vi "RPT_Convert Results.vi"(9 "disabled index (col)":i32, 10 "Results IN":T1 {"Resistor 2" format="%.1f"; "Drain" format="%.3f"; "Resistor" format="%.1f"; "Fill" format="%.3f"}) -> (2 "Report OUt":string[][](array[string]), 3 "ATP Table":string[][](array[string]))   [LabVIEW 2024]
uses:
  Control Definitions/Def Results3.ctl
  Control Definitions/Def_ATPStatus.ctl
  Control Definitions/Def Results.ctl
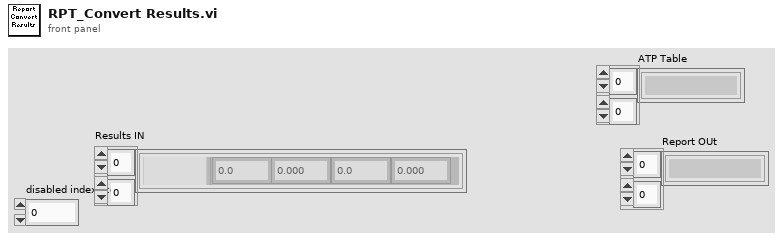
[diagram p1: front panel]
types:
  T1 = typedef "Def Results.ctl" = T2[][]
  T2 = typedef "Def Results3.ctl" = cluster{"Fill":dbl, "Status":T3, "Resistor":dbl, "Drain":dbl, "Resistor 2":dbl}
  T3 = typedef "Def_ATPStatus.ctl" = i16
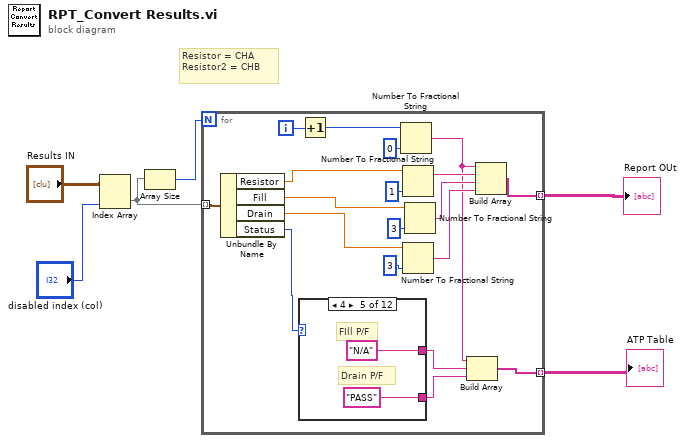
[diagram p0: block diagram]
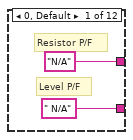
[diagram p2: hidden frame]
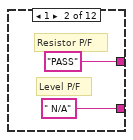
[diagram p3: hidden frame]
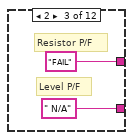
[diagram p4: hidden frame]
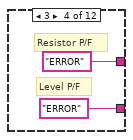
[diagram p5: hidden frame]
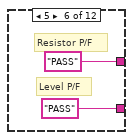
[diagram p6: hidden frame]
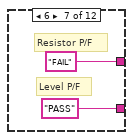
[diagram p7: hidden frame]
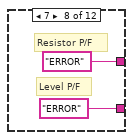
[diagram p8: hidden frame]
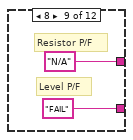
[diagram p9: hidden frame]
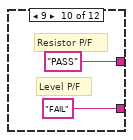
[diagram p10: hidden frame]
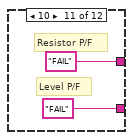
[diagram p11: hidden frame]
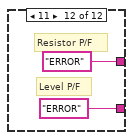
[diagram p12: hidden frame]
diagram:
  # "Resistor = CHA\nResistor2 = CHB"
  n1 = Index Array(array="Results IN", index (col)="disabled index (col)") -> (element=w5:T2[])  [unwired: 1 in]
  n2 = Array Size(array=w5) -> (size(s)=w4:i32)
  n3 = for {
    N: w4 -> [_]
    tunnel: w5 -> [w15] mode=indexing
    tunnel: [w19] -> w6 mode=indexing
    tunnel: [w8] -> w1 mode=indexing
    i -> [w18]
    n4 = Unbundle By Name(w15) -> ("Resistor"=w14:dbl, "Fill"=w13:dbl, "Drain"=w12:dbl, "Status"=w11:T3)
    n5 = case shown="4" w11 {
      tunnel: ["N/A" "PASS" "FAIL" "ERROR" "N/A" "PASS" "FAIL" "ERROR" "N/A" "PASS" "FAIL" "ERROR"] -> w10
      tunnel: [" N/A" " N/A" " N/A" "ERROR" "PASS" "PASS" "PASS" "ERROR" "FAIL" "FAIL" "FAIL" "ERROR"] -> w9
      frame 0, Default {
        # "Resistor P/F"
        # "Level P/F"
      }
      frame 1 {
        # "Resistor P/F"
        # "Level P/F"
      }
      frame 2 {
        # "Resistor P/F"
        # "Level P/F"
      }
      frame 3 {
        # "Resistor P/F"
        # "Level P/F"
      }
      frame 4 {
        # "FIll P/F"
        # "Drain P/F"
      }
      frame 5 {
        # "Resistor P/F"
        # "Level P/F"
      }
      frame 6 {
        # "Resistor P/F"
        # "Level P/F"
      }
      frame 7 {
        # "Resistor P/F"
        # "Level P/F"
      }
      frame 8 {
        # "Resistor P/F"
        # "Level P/F"
      }
      frame 9 {
        # "Resistor P/F"
        # "Level P/F"
      }
      frame 10 {
        # "Resistor P/F"
        # "Level P/F"
      }
      frame 11 {
        # "Resistor P/F"
        # "Level P/F"
      }
    }
    n6 = Increment(x=w18) -> (x+1=w16:i32)
    n7 = Number To Fractional String(number=w16, precision (6)=i16 0) -> (F-format string=w7:string)  [unwired: 2 in]
    n8 = Number To Fractional String(number=w14, precision (6)=i16 1) -> (F-format string=w22:string)  [unwired: 2 in]
    n9 = Number To Fractional String(number=w12, precision (6)=i16 3) -> (F-format string=w20:string)  [unwired: 2 in]
    n10 = Number To Fractional String(number=w13, precision (6)=i16 3) -> (F-format string=w21:string)  [unwired: 2 in]
    n11 = Build Array(w7, w10, w9) -> (w8:string[])
    n12 = Build Array(w7, w22, w21, w20) -> (w19:string[])
  }
  "Report OUt" <- w6
  "ATP Table" <- w1
